vi "Read min record length (100 samples).vi"(8 "error in (no error)":errorcluster, 11 "Configure Acquisition Record Msg in":refnum<class "Configure Acquisition Record Msg.lvclass">) -> (0 "error out":errorcluster, 2 "min record length (100 samples)":i32=100, 3 "Configure Acquisition Record Msg out":refnum<class "Configure Acquisition Record Msg.lvclass">)   [LabVIEW 2016, in "CS++Scope.lvlib" / "Configure Acquisition Record Msg.lvclass"]
uses:
  Configure Acquisition Record Msg.lvclass
  Configure Acquisition Record Msg.lvclass/Configure Acquisition Record Msg.ctl
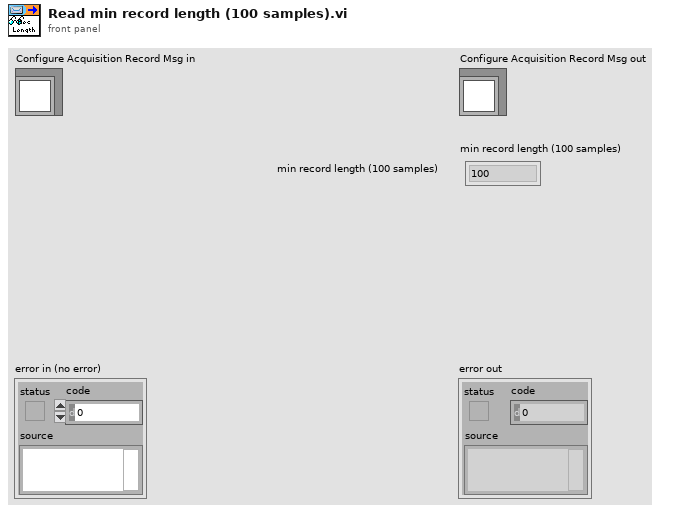
[diagram p1: front panel]
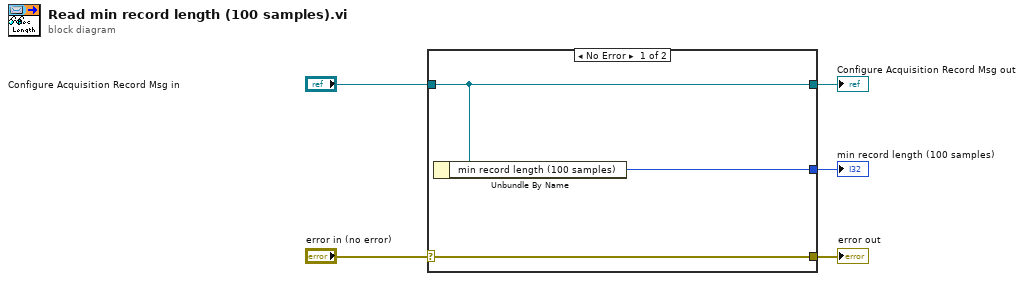
[diagram p0: block diagram]
diagram:
  n1 = case shown="No Error" "error in (no error)" {
    selector: "error in (no error)" -> [w8 w9]
    tunnel: [w8 w9] -> w4
    tunnel: [w7 w10] -> w2
    tunnel: "Configure Acquisition Record Msg in" -> [w7 w10]
    tunnel: [w6 _] -> w1
    frame No Error {
      n2 = Unbundle By Name(w7) -> ("min record length (100 samples)"=w6:i32)
    }
    frame Error {
    }
  }
  "error out" <- w4
  "Configure Acquisition Record Msg out" <- w2
  "min record length (100 samples)" <- w1
